vi "Shooter Control.vi"(0 "Shooter Wheel On?":bool, 1 "Fire":bool, 4 "Rotate Tweak":dbl(slide) scale=-1.0..1.0, 5 "Harvester Axis":dbl(slide) scale=-1.0..1.0, 7 "Shooter Arm Level":i32) -> ()   [LabVIEW 2015]
uses:
  <vilib>/Rock Robotics/Network Tables/NT Read Number.vi
  Robot Global Data.vi
panel:
  in  "Shooting Time for Feeder":u64=750
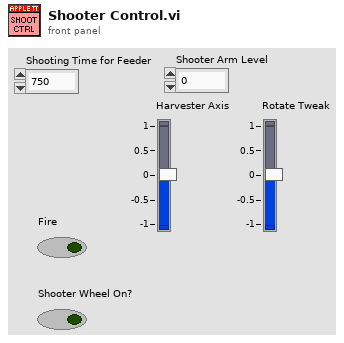
[diagram p1: front panel]
types:
  T1 = typedef "WPI_MotorControlDeviceRef.ctl" = cluster{"DeviceStatus":errorcluster, "Type":T2, "PWM":cluster{"PWM Channel":T3, "DeadBand":T4}, "CAN":cluster{"Device Number":u8, "Control Mode":T5, "Semaphore":T6, "Max Vout":dbl, "TalonSRX Control Mode":T7}, "Invert":bool}
  T2 = typedef "WPI_MotorControlType.ctl" = enum16{"PWM", "CAN", "CANTalonSRX"}
  T3 = typedef "FPGA_DIOPWMChannel.ctl" = enum8{"PWM 0", "PWM 1", "PWM 2", "PWM 3", "PWM 4", "PWM 5", "PWM 6", "PWM 7", "PWM 8", "PWM 9", "PWM MXP 0", "PWM MXP 1", "PWM MXP 2", "PWM MXP 3", "PWM MXP 4", "PWM MXP 5", "PWM MXP 6", "PWM MXP 7", "PWM MXP 8", "PWM MXP 9", "Invalid"}
  T4 = typedef "WPI_PWMDeadband.ctl" = cluster{"Name":string, "maxPositivePwm":i32, "minPositivePwm":i32, "centerPwm":i32, "maxNegativePwm":i32, "minNegativePwm":i32, "angularRange":u16}
  T5 = typedef "WPI_CANJaguar_ControlMode.ctl" = enum8{"Percent VBus", "Current", "Speed", "Position", "Voltage"}
  T6 = typedef "Semaphore RefNum" = refnum<k1>
  T7 = typedef "WPI_CANTalonSRX_APIControlMode.ctl" = enum8{"Percent VBus", "Speed", "Position", "Slave", "Unchanged / Invalid", "Voltage Compensation", "Current", "Motion Profile"}
  T8 = typedef "WPI_DigitalInputDevRef.ctl" = cluster{"DevStatus":errorcluster, "DIO Channel":T9}
  T9 = typedef "FPGA_DIOChannel.ctl" = enum8{"DIO 0", "DIO 1", "DIO 2", "DIO 3", "DIO 4", "DIO 5", "DIO 6", "DIO 7", "DIO 8", "DIO 9", "DIO MXP 0", "DIO MXP 1", "DIO MXP 2", "DIO MXP 3", "DIO MXP 4", "DIO MXP 5", "DIO MXP 6", "DIO MXP 7", "DIO MXP 8", "DIO MXP 9", "DIO MXP 10", "DIO MXP 11", "DIO MXP 12", "DIO MXP 13", "DIO MXP 14", "DIO MXP 15", "Invalid"}
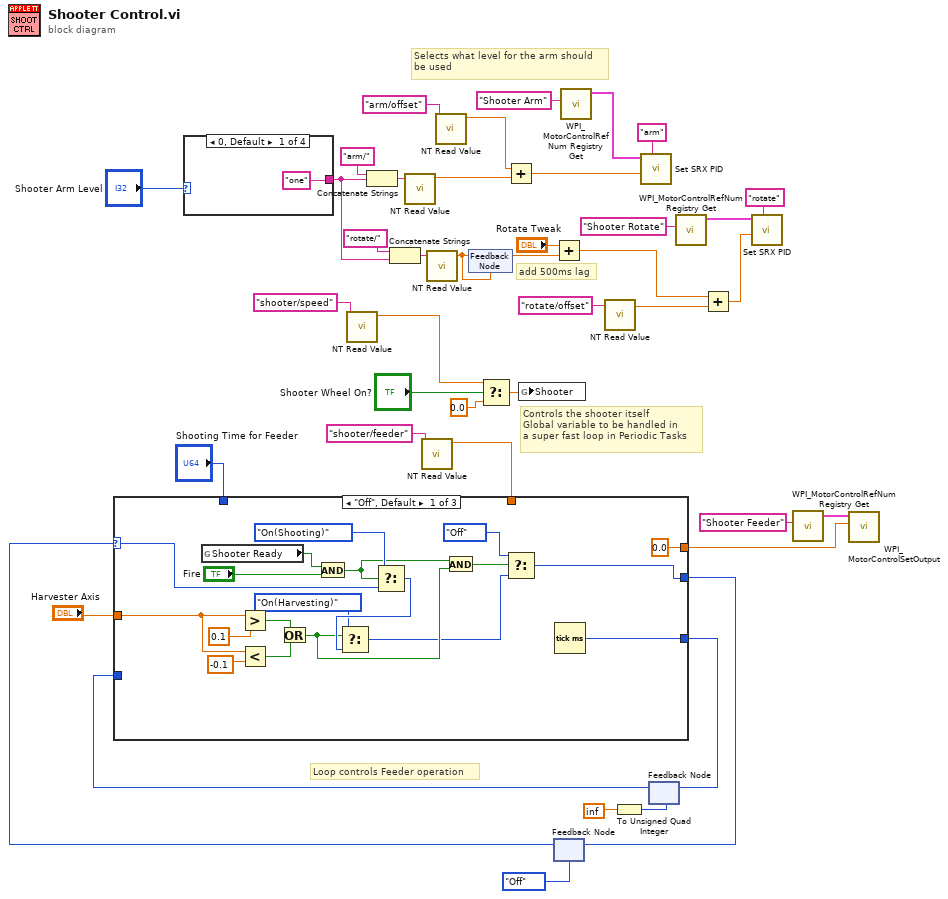
[diagram p0: block diagram]
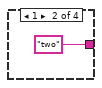
[diagram p2: hidden frame]
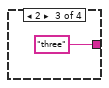
[diagram p3: hidden frame]
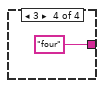
[diagram p4: hidden frame]
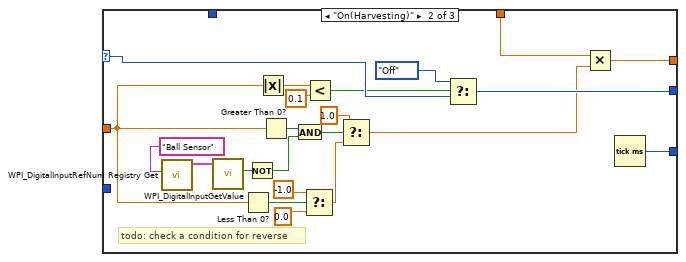
[diagram p5: hidden frame]
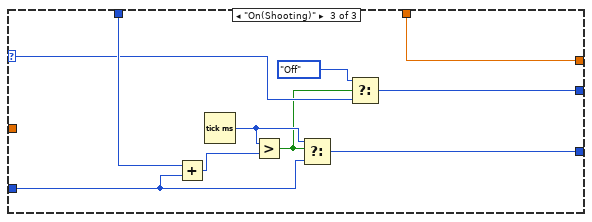
[diagram p6: hidden frame]
diagram:
  # "add 500ms lag"
  # "Controls the shooter itself\nGlobal variable to be handled in\na super fast loop in Periodic Tasks"
  # "Selects what level for the arm should\nbe used"
  # "Loop controls Feeder operation"
  n1 = case shown="0, Default" "Shooter Arm Level" {
    tunnel: ["one" ("Name") "two" ("Name") "three" ("Name") "four" ("Name")] -> w9
    frame 0, Default {
    }
    frame 1 {
    }
    frame 2 {
    }
    frame 3 {
    }
  }
  n2 = call-poly <vilib>:"NT Read Value.vi"("Name"="shooter/speed") -> ("Numeric"=w19:dbl)  [unwired: 9 in, 1 out]
  n3 = Concatenate Strings("arm/" ("Name"), w9) -> (w13:string)
  n4 = Concatenate Strings("rotate/" ("Name"), w9) -> (w11:string)
  n5 = call-poly <vilib>:"NT Read Value.vi"("Name"=w13) -> ("Numeric"=w26:dbl)  [unwired: 9 in, 1 out]
  n6 = call-poly <vilib>:"NT Read Value.vi"("Name"="shooter/feeder") -> ("Numeric"=w3:dbl)  [unwired: 9 in, 1 out]
  n7 = call-poly <vilib>:"NT Read Value.vi"("Name"=w11) -> ("Numeric"=w2:dbl)  [unwired: 9 in, 1 out]
  n8 = call-poly <vilib>:"NT Read Value.vi"("Name"="arm/offset") -> ("Numeric"=w27:dbl)  [unwired: 9 in, 1 out]
  n9 = feedback-in #1(w2) -> ()
  n10 = feedback #1(w2) -> (w5:dbl)
  n11 = Select(t=w19, s="Shooter Wheel On?", f=0.0) -> (s? t:f=w21:dbl)
  n12 = Add(x=w27, y=w26) -> (x+y=w25:dbl)
  n13 = global write "Robot Global Data.vi" "Shooter"(w21) -> ()
  n14 = Add(x="Rotate Tweak", y=w5) -> (x+y=w7:dbl)
  n15 = feedback #2(enum16{"Off", "On(Shooting)", "On(Harvesting)"}."Off") -> (w38:enum16{"Off", "On(Shooting)", "On(Harvesting)"})
  n16 = call <vilib>:"WPI_MotorControlRefNum Registry Get.vi"("refnum name"="Shooter Arm") -> ("MotorControlDevRef"=w22:T1)  [unwired: 9 in, 1 out]
  n17 = call-poly <vilib>:"NT Read Value.vi"("Name"="rotate/offset") -> ("Numeric"=w17:dbl)  [unwired: 9 in, 1 out]
  n18 = To Unsigned Quad Integer(1:inf) -> (0:w32:u64)
  n19 = call "Set SRX PID.vi"("subsystem"="arm", "Setpoint"=w25, "CAN Talon SRX Ref"=w22) -> ()  [unwired: 8 in, 1 out]
  n20 = feedback #3(w32) -> (w34:u64)
  n21 = case shown="\"Off\", Default" w38 {
    selector: w38 -> [w61 w85 w91]
    tunnel: [w53 w86 w89] -> w36
    tunnel: [w52 w67 w93] -> w35
    tunnel: w34 -> [_ _ w94]
    tunnel: "Shooting Time for Feeder" -> [_ _ w97]
    tunnel: [0.0 w79 w88] -> w31
    tunnel: "Harvester Axis" -> [w50 w72 _]
    tunnel: w3 -> [_ w66 w88]
    frame "Off", Default {
      n22 = global read "Robot Global Data.vi" "Shooter Ready"() -> (w49:bool)
      n23 = Greater?(x=w50, y=0.1) -> (0:w64:bool)
      n24 = Less?(x=w50, y=-0.1) -> (x < y?=w65:bool)
      n25 = Or(x=w64, y=w65) -> (x .or. y?=w57:bool)
      n26 = And(x=w49, y="Fire") -> (x .and. y?=w47:bool)
      n27 = Select(t=enum16{"Off", "On(Shooting)", "On(Harvesting)"}."On(Shooting)", s=w47, f=w61) -> (s? t:f=w59:enum16{"Off", "On(Shooting)", "On(Harvesting)"})
      n28 = Select(t=enum16{"Off", "On(Shooting)", "On(Harvesting)"}."On(Harvesting)", s=w57, f=w59) -> (s? t:f=w55:enum16{"Off", "On(Shooting)", "On(Harvesting)"})
      n29 = And(x=w47, y=w57) -> (x .and. y?=w56:bool)
      n30 = Select(t=enum16{"Off", "On(Shooting)", "On(Harvesting)"}."Off", s=w56, f=w55) -> (s? t:f=w53:enum16{"Off", "On(Shooting)", "On(Harvesting)"})
      n31 = Tick Count (ms)() -> (millisecond timer value=w52:u32)
    }
    frame "On(Harvesting)" {
      # "todo: check a condition for reverse"
      n32 = call <vilib>:"WPI_DigitalInputRefNum Registry Get.vi"("refnum name"="Ball Sensor") -> ("DigitalInputDevRef"=w84:T8)  [unwired: 9 in, 1 out]
      n33 = call <vilib>:"WPI_DigitalInputGetValue.vi"("DigitalInputDevRef"=w84) -> ("Value"=w77:bool)  [unwired: 8 in, 2 out]
      n34 = Less Than 0?(x=w72) -> (x < 0?=w70:bool)
      n35 = Not(x=w77) -> (.not. x?=w76:bool)
      n36 = Absolute Value(x=w72) -> (abs(x)=w82:dbl)
      n37 = Greater Than 0?(x=w72) -> (x > 0?=w78:bool)
      n38 = And(x=w78, y=w76) -> (x .and. y?=w75:bool)
      n39 = Select(t=-1.0, s=w70, f=0.0) -> (s? t:f=w68:dbl)
      n40 = Less?(x=w82, y=0.1) -> (x < y?=w80:bool)
      n41 = Select(t=1.0, s=w75, f=w68) -> (s? t:f=w73:dbl)
      n42 = Select(t=enum16{"Off", "On(Shooting)", "On(Harvesting)"}."Off", s=w80, f=w85) -> (s? t:f=w86:enum16{"Off", "On(Shooting)", "On(Harvesting)"})
      n43 = Multiply(x=w66, y=w73) -> (x*y=w79:dbl)
      n44 = Tick Count (ms)() -> (millisecond timer value=w67:u32)
    }
    frame "On(Shooting)" {
      n45 = Add(x=w97, y=w94) -> (x+y=w96:u64)
      n46 = Tick Count (ms)() -> (millisecond timer value=w95:u32)
      n47 = Greater?(x=w95, y=w96) -> (0:w90:bool)
      n48 = Select(t=w95, s=w90, f=w94) -> (s? t:f=w93:u64)
      n49 = Select(t=enum16{"Off", "On(Shooting)", "On(Harvesting)"}."Off", s=w90, f=w91) -> (s? t:f=w89:enum16{"Off", "On(Shooting)", "On(Harvesting)"})
    }
  }
  n50 = feedback-in #2(w36) -> ()
  n51 = feedback-in #3(w35) -> ()
  n52 = call <vilib>:"WPI_MotorControlRefNum Registry Get.vi"("refnum name"="Shooter Rotate") -> ("MotorControlDevRef"=w16:T1)  [unwired: 9 in, 1 out]
  n53 = Add(x=w7, y=w17) -> (x+y=w15:dbl)
  n54 = call "Set SRX PID.vi"("subsystem"="rotate", "Setpoint"=w15, "CAN Talon SRX Ref"=w16) -> ()  [unwired: 8 in, 1 out]
  n55 = call <vilib>:"WPI_MotorControlRefNum Registry Get.vi"("refnum name"="Shooter Feeder") -> ("MotorControlDevRef"=w40:T1)  [unwired: 9 in, 1 out]
  n56 = call <vilib>:"WPI_MotorControlSetOutput.vi"("Output"=w31, "MotorControlDevRef"=w40) -> ()  [unwired: 7 in, 3 out]
